vi "Query Trace Data.vi"(8 "error in (no error)":errorcluster, 10 "Trace Number":u8=1, 11 "VNA-ENA in":refnum<class "VNA-ENA.lvclass">) -> (0 "error out":errorcluster, 1 "Data":dbl[](array[numeric]), 2 "Frequency":dbl[](array[numeric]), 3 "VNA-ENA out":refnum<class "VNA-ENA.lvclass">)   [LabVIEW 2020, in "VNA-ENA.lvclass"]
doc: "Query the active trace data.\nIt returns both x and y data"
uses:
  VNA-ENA.lvclass
  C:/Sandbox/Git_Sandbox/WiSpry Test Framework source code (LV20)/WiSpry Test Framework/Instruments/Instrument.lvclass
  Instrument.lvclass/Instrument.ctl
  Instrument.lvclass
  <instrlib>/Agilent ENA Series/Agilent ENA Series.lvlib
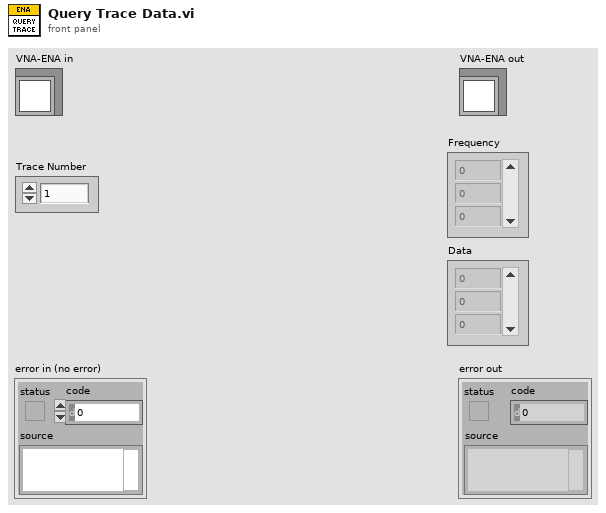
[diagram p1: front panel]
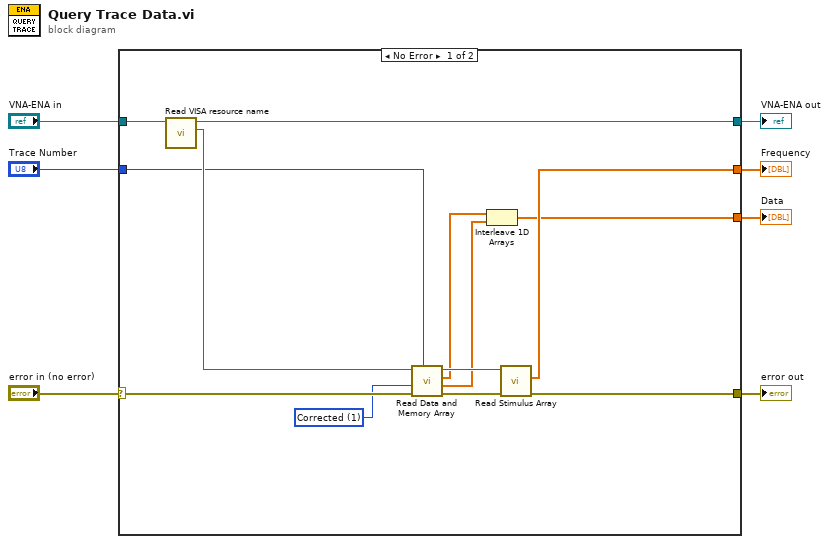
[diagram p0: block diagram]
diagram:
  n1 = case shown="No Error" "error in (no error)" {
    selector: "error in (no error)" -> [w19 w22]
    tunnel: [w14 w22] -> w6
    tunnel: [w17 w21] -> w5
    tunnel: "VNA-ENA in" -> [w20 w21]
    tunnel: [w13 _] -> w3
    tunnel: [w10 _] -> w2
    tunnel: "Trace Number" -> [w9 _]
    frame No Error {
      w8 = u16 1 items=["Formatted", "Corrected"] ("Correction (0: Data)")
      n2 = call "Read VISA resource name.vi"("Instrument in"=w20) -> ("VISA resource name"=w18:refnum<visa-resource-name>, "Instrument out"=w17:refnum<class "VNA-ENA.lvclass">)  [unwired: 9 in]
      n3 = call <instrlib>:"Read Data and Memory Array.vi"("Channel (1)"=w9, "error in (no error)"=w19, "Correction (0: Data)"=w8, "VISA resource name"=w18) -> ("error out"=w15:errorcluster, "Secondary / Imaginary"=w12:dbl[], "Primary / Real"=w11:dbl[], "VISA resource name out"=w16:refnum<visa-resource-name>)  [unwired: 4 in]
      n4 = Interleave 1D Arrays(w11, w12) -> (w10:dbl[])
      n5 = call <instrlib>:"Read Stimulus Array.vi"("error in (no error)"=w15, "VISA resource name"=w16) -> ("error out"=w14:errorcluster, "Stimulus Data"=w13:dbl[])  [unwired: 7 in, 1 out]
    }
    frame Error {
    }
  }
  "error out" <- w6
  "VNA-ENA out" <- w5
  "Data" <- w2
  "Frequency" <- w3
